vi "Read Size.vi"(9 "IOName in":refnum<class "IOName.lvclass">) -> (3 "IOName out":refnum<class "IOName.lvclass">, 4 "Size":T1)   [LabVIEW 2014, in "Raspberry Pi Compatible Compiler for LabVIEW.lvlib" / "IOName.lvclass"]
uses:
  IOName.lvclass
  <vilib>/Utility/miscctls.llb/LVBoundsTypeDef.ctl
  IOName.lvclass/IOName.ctl
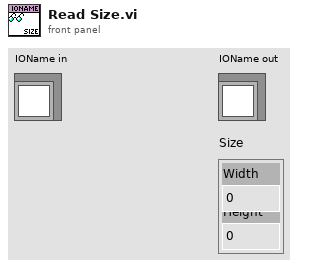
[diagram p1: front panel]
types:
  T1 = typedef "LVBoundsTypeDef.ctl" = cluster{"Width":u32, "Height":u32}
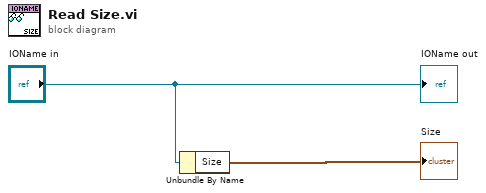
[diagram p0: block diagram]
diagram:
  n1 = Unbundle By Name("IOName in") -> ("Size"=→"Size":T1)
  "IOName out" <- "IOName in"
